vi "Read Auto Drive constants minus Auto Transmission.vi"(8 "error in (no error)":errorcluster) -> (0 "error out":errorcluster, 3 "Auto Drive Constants":T1)   [LabVIEW 2013]
uses:
  Drive auto constants.ctl
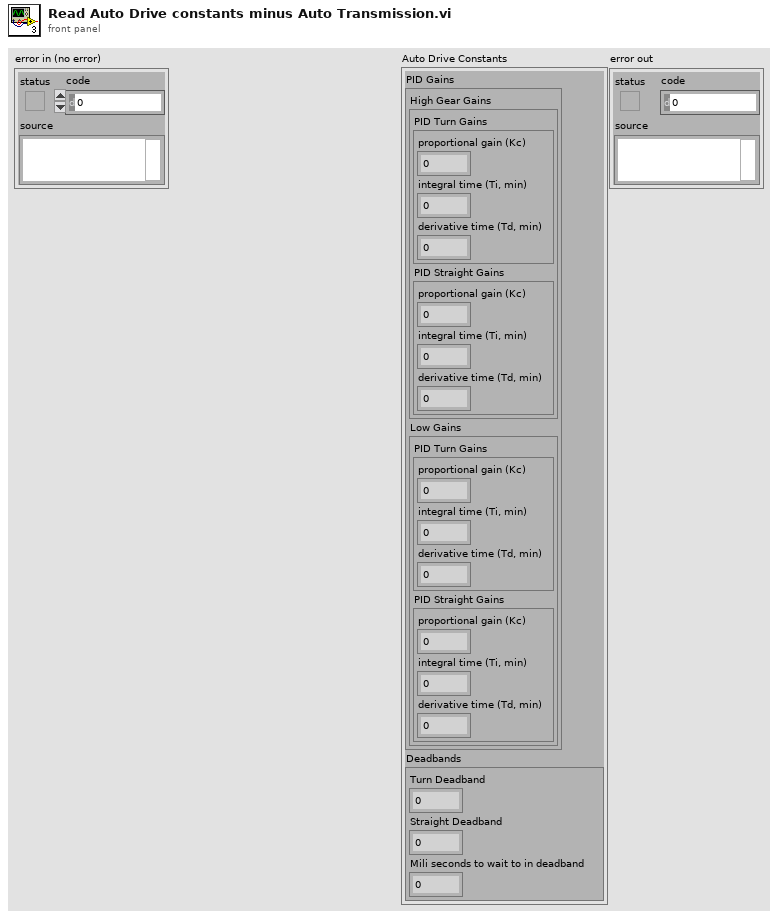
[diagram p1: front panel]
types:
  T1 = typedef "Drive auto constants.ctl" = cluster{"PID Gains":cluster{"High Gear Gains":cluster{"PID Turn Gains":cluster{"proportional gain (Kc)":dbl, "integral time (Ti, min)":dbl, "derivative time (Td, min)":dbl}, "PID Straight Gains":cluster{"proportional gain (Kc)":dbl, "integral time (Ti, min)":dbl, "derivative time (Td, min)":dbl}}, "Low Gains":cluster{"PID Turn Gains":cluster{"proportional gain (Kc)":dbl, "integral time (Ti, min)":dbl, "derivative time (Td, min)":dbl}, "PID Straight Gains":cluster{"proportional gain (Kc)":dbl, "integral time (Ti, min)":dbl, "derivative time (Td, min)":dbl}}}, "Deadbands":cluster{"Turn Deadband":dbl, "Straight Deadband":dbl, "Mili seconds to wait to in deadband":u32}}
  T2 = cluster{"High Gear Gains":cluster{"PID Turn Gains":cluster{"proportional gain (Kc)":dbl, "integral time (Ti, min)":dbl, "derivative time (Td, min)":dbl}, "PID Straight Gains":cluster{"proportional gain (Kc)":dbl, "integral time (Ti, min)":dbl, "derivative time (Td, min)":dbl}}, "Low Gains":cluster{"PID Turn Gains":cluster{"proportional gain (Kc)":dbl, "integral time (Ti, min)":dbl, "derivative time (Td, min)":dbl}, "PID Straight Gains":cluster{"proportional gain (Kc)":dbl, "integral time (Ti, min)":dbl, "derivative time (Td, min)":dbl}}}
  T3 = cluster{"Turn Deadband":dbl, "Straight Deadband":dbl, "Mili seconds to wait to in deadband":u32}
  T4 = cluster{"PID Turn Gains":cluster{"proportional gain (Kc)":dbl, "integral time (Ti, min)":dbl, "derivative time (Td, min)":dbl}, "PID Straight Gains":cluster{"proportional gain (Kc)":dbl, "integral time (Ti, min)":dbl, "derivative time (Td, min)":dbl}}
  T5 = cluster{"proportional gain (Kc)":dbl, "integral time (Ti, min)":dbl, "derivative time (Td, min)":dbl}
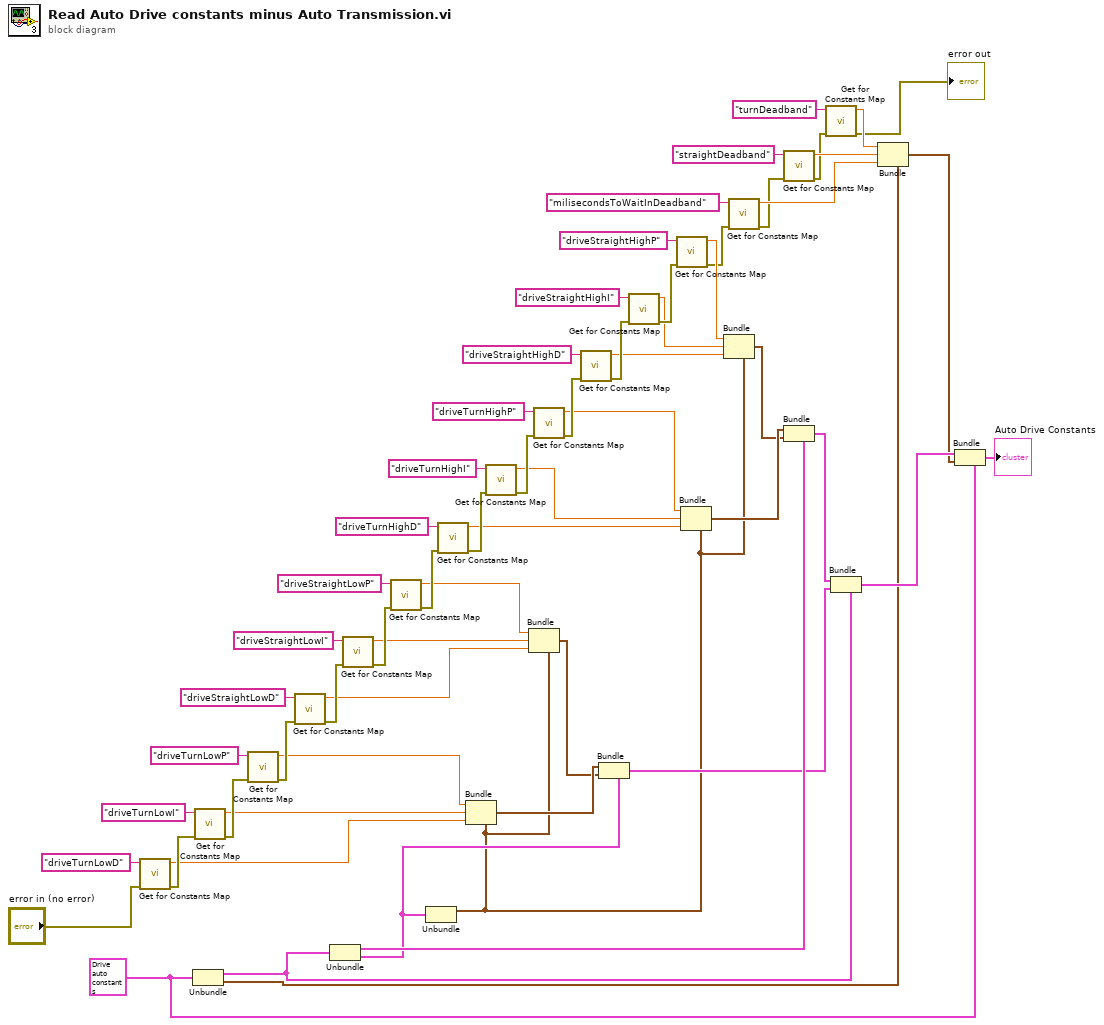
[diagram p0: block diagram]
diagram:
  w38 = T1 {"PID Gains"={"High Gear Gains"={"PID Turn Gains"={"proportional gain (Kc)"=0.0, "integral time (Ti, min)"=0.0, "derivative time (Td, min)"=0.0}, "PID Straight Gains"={"proportional gain (Kc)"=0.0, "integral time (Ti, min)"=0.0, "derivative time (Td, min)"=0.0}}, "Low Gains"={"PID Turn Gains"={"proportional gain (Kc)"=0.0, "integral time (Ti, min)"=0.0, "derivative time (Td, min)"=0.0}, "PID Straight Gains"={"proportional gain (Kc)"=0.0, "integral time (Ti, min)"=0.0, "derivative time (Td, min)"=0.0}}}, "Deadbands"={"Turn Deadband"=0.0, "Straight Deadband"=0.0, "Mili seconds to wait to in deadband"=0}} ("Drive Constants")
  n1 = call "Get for Constants Map.vi"("error in (no error)"="error in (no error)", "Constant Name"="driveTurnLowD") -> ("error out"=w44:errorcluster, "Value"=w25:dbl)  [unwired: 7 in, 1 out]
  n2 = Unbundle(w38) -> ("PID Gains"=w36:T2, "Deadbands"=w14:T3)
  n3 = call "Get for Constants Map.vi"("error in (no error)"=w44, "Constant Name"="driveTurnLowI") -> ("error out"=w45:errorcluster, "Value"=w26:dbl)  [unwired: 7 in, 1 out]
  n4 = call "Get for Constants Map.vi"("error in (no error)"=w45, "Constant Name"="driveTurnLowP") -> ("error out"=w61:errorcluster, "Value"=w27:dbl)  [unwired: 7 in, 1 out]
  n5 = call "Get for Constants Map.vi"("error in (no error)"=w61, "Constant Name"="driveStraightLowD") -> ("error out"=w60:errorcluster, "Value"=w16:dbl)  [unwired: 7 in, 1 out]
  n6 = Unbundle(w36) -> ("High Gear Gains"=w35:T4, "Low Gains"=w28:T4)
  n7 = call "Get for Constants Map.vi"("error in (no error)"=w60, "Constant Name"="driveStraightLowI") -> ("error out"=w59:errorcluster, "Value"=w17:dbl)  [unwired: 7 in, 1 out]
  n8 = call "Get for Constants Map.vi"("error in (no error)"=w59, "Constant Name"="driveStraightLowP") -> ("error out"=w58:errorcluster, "Value"=w18:dbl)  [unwired: 7 in, 1 out]
  n9 = Unbundle(w28) -> ("PID Turn Gains"=w19:T5)  [unwired: 1 out]
  n10 = call "Get for Constants Map.vi"("error in (no error)"=w58, "Constant Name"="driveTurnHighD") -> ("error out"=w57:errorcluster, "Value"=w32:dbl)  [unwired: 7 in, 1 out]
  n11 = Bundle(cluster=w19, "proportional gain (Kc)"=w27, "integral time (Ti, min)"=w26, "derivative time (Td, min)"=w25) -> (w24:T5)
  n12 = call "Get for Constants Map.vi"("error in (no error)"=w57, "Constant Name"="driveTurnHighI") -> ("error out"=w56:errorcluster, "Value"=w33:dbl)  [unwired: 7 in, 1 out]
  n13 = Bundle(cluster=w19, "proportional gain (Kc)"=w18, "integral time (Ti, min)"=w17, "derivative time (Td, min)"=w16) -> (w15:T5)
  n14 = call "Get for Constants Map.vi"("error in (no error)"=w56, "Constant Name"="driveTurnHighP") -> ("error out"=w55:errorcluster, "Value"=w34:dbl)  [unwired: 7 in, 1 out]
  n15 = call "Get for Constants Map.vi"("error in (no error)"=w55, "Constant Name"="driveStraightHighD") -> ("error out"=w54:errorcluster, "Value"=w29:dbl)  [unwired: 7 in, 1 out]
  n16 = Bundle(cluster=w28, "PID Turn Gains"=w24, "PID Straight Gains"=w15) -> (w20:T4)
  n17 = call "Get for Constants Map.vi"("error in (no error)"=w54, "Constant Name"="driveStraightHighI") -> ("error out"=w53:errorcluster, "Value"=w30:dbl)  [unwired: 7 in, 1 out]
  n18 = call "Get for Constants Map.vi"("error in (no error)"=w53, "Constant Name"="driveStraightHighP") -> ("error out"=w11:errorcluster, "Value"=w31:dbl)  [unwired: 7 in, 1 out]
  n19 = Bundle(cluster=w19, "proportional gain (Kc)"=w34, "integral time (Ti, min)"=w33, "derivative time (Td, min)"=w32) -> (w23:T5)
  n20 = Bundle(cluster=w19, "proportional gain (Kc)"=w31, "integral time (Ti, min)"=w30, "derivative time (Td, min)"=w29) -> (w22:T5)
  n21 = call "Get for Constants Map.vi"("error in (no error)"=w11, "Constant Name"="milisecondsToWaitInDeadband") -> ("error out"=w9:errorcluster, "Value"=w10:dbl)  [unwired: 7 in, 1 out]
  n22 = call "Get for Constants Map.vi"("error in (no error)"=w9, "Constant Name"="straightDeadband") -> ("error out"=w6:errorcluster, "Value"=w8:dbl)  [unwired: 7 in, 1 out]
  n23 = Bundle(cluster=w35, "PID Turn Gains"=w23, "PID Straight Gains"=w22) -> (w21:T4)
  n24 = call "Get for Constants Map.vi"("error in (no error)"=w6, "Constant Name"="turnDeadband") -> ("error out"=→"error out":errorcluster, "Value"=w7:dbl)  [unwired: 7 in, 1 out]
  n25 = Bundle(cluster=w36, "High Gear Gains"=w21, "Low Gains"=w20) -> (w37:T2)
  n26 = Bundle(cluster=w14, "Turn Deadband"=w7, "Straight Deadband"=w8, "Mili seconds to wait to in deadband"=w10) -> (w13:T3)
  n27 = Bundle(cluster=w38, "PID Gains"=w37, "Deadbands"=w13) -> (→"Auto Drive Constants":T1)
